vi "Report - Add Section Header.vi"(0 "report in":refnum<class "NI_report.lvclass">, 1 "Heading Size":enum16{"h1", "h2", "h3"}(ring), 5 "Heading Text":string, 11 "error in (no error)":errorcluster) -> (4 "report out":refnum<class "NI_report.lvclass">, 15 "error out":errorcluster)   [LabVIEW 2010]
uses:
  <vilib>/Utility/NIReport.llb/NI_report.lvclass
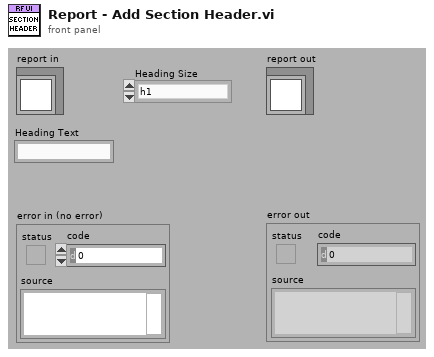
[diagram p1: front panel]
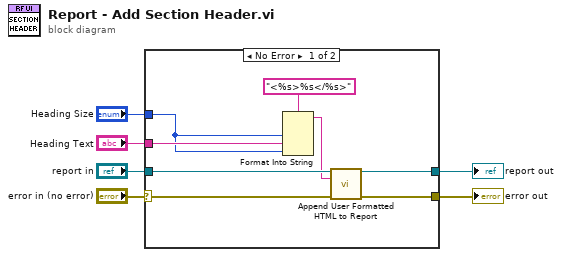
[diagram p0: block diagram]
diagram:
  n1 = case shown="No Error" "error in (no error)" {
    selector: "error in (no error)" -> [w13 w15]
    tunnel: "report in" -> [w14 w16]
    tunnel: "Heading Text" -> [w11 _]
    tunnel: [w8 w15] -> w3
    tunnel: [w9 w16] -> w2
    tunnel: "Heading Size" -> [w7 _]
    frame No Error {
      n2 = Format Into String(format string="<%s>%s</%s>", w7, w11, w7) -> (resulting string=w10:string)  [unwired: 2 in, 1 out]
      n3 = call-dynamic "Append User Formatted HTML to Report.vi"("report in"=w14, "HTML text"=w10, "error in (no error)"=w13) -> ("report out"=w9:refnum<class "NI_report.lvclass">, "error out"=w8:errorcluster)  [unwired: 11 in]
    }
    frame Error {
    }
  }
  "report out" <- w2
  "error out" <- w3
